vi "TimerOnDelay.vi"(10 "Time Delay":u32, 11 "Input":bool) -> (3 "Output":bool)   [LabVIEW 2016]
doc: "Output becomes true Time Limit ms after Input becomes true and stays true"
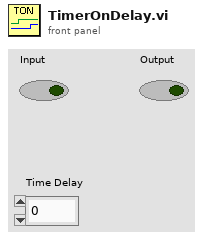
[diagram p1: front panel]
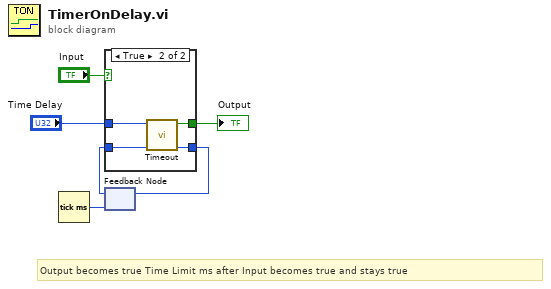
[diagram p0: block diagram]
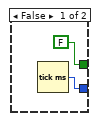
[diagram p2: hidden frame]
diagram:
  # "Output becomes true Time Limit ms after Input becomes true and stays true"
  n1 = Tick Count (ms)() -> (millisecond timer value=w4:u32)
  n2 = feedback #1(w4) -> (w2:u32)
  n3 = case shown="True" "Input" {
    tunnel: [FALSE ("Output") w9] -> w5
    tunnel: [w7 w11] -> w3
    tunnel: w2 -> [_ w12]
    tunnel: "Time Delay" -> [_ w10]
    frame False {
      n4 = Tick Count (ms)() -> (millisecond timer value=w7:u32)
    }
    frame True {
      n5 = call "Timeout.vi"("Start Time In"=w12, "Time Limit (ms)"=w10) -> ("Start Time Out"=w11:u32, "Timeout"=w9:bool)  [unwired: 8 in]
    }
  }
  "Output" <- w5
  n6 = feedback-in #1(w3) -> ()
